vi "WriteValueToQueueDisplay.vi"(8 "error in (no error)":errorcluster, 11 "XuLyStringUART in":refnum<class "XuLyStringUART.lvclass">) -> (0 "error out":errorcluster, 3 "XuLyStringUART out":refnum<class "XuLyStringUART.lvclass">)   [LabVIEW 2017, in "LibraryGcode.lvlib" / "XuLyStringUART.lvclass"]
uses:
  XuLyStringUART.lvclass
  control/UartCmdQueueUpdate.ctl
panel:
  in  "Command":T1
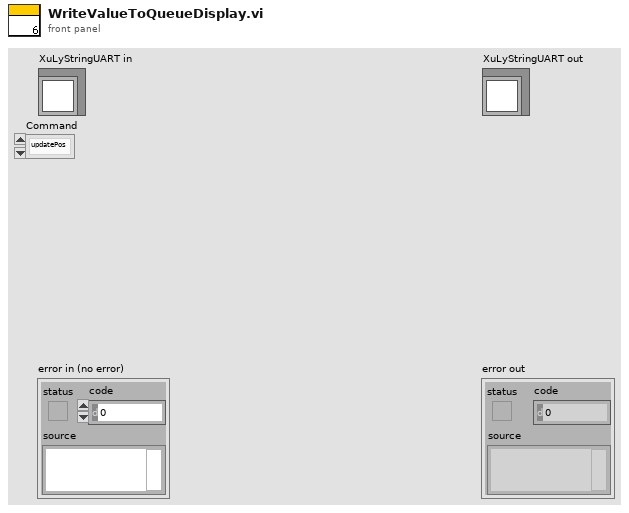
[diagram p1: front panel]
types:
  T1 = typedef "UartCmdQueueUpdate.ctl" = enum16{"updatePos", "UpdateConfigAccel", "UpdateConfigFeed", "UpdateConfigUnit", "UpdateConfigStartAccel"}
  T2 = cluster{"Command":T1, "POS":cluster{"X":dbl, "Y":dbl, "Z":dbl}, "DEGREES":cluster{"X":dbl, "Y":dbl}}
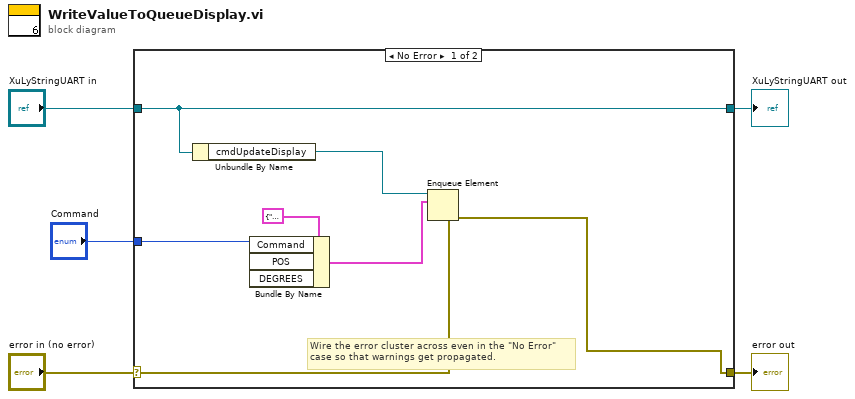
[diagram p0: block diagram]
diagram:
  n1 = case shown="No Error" "error in (no error)" {
    selector: "error in (no error)" -> [w11 w14]
    tunnel: [w10 w14] -> w4
    tunnel: [w12 w13] -> w2
    tunnel: "XuLyStringUART in" -> [w12 w13]
    tunnel: "Command" -> [w6 _]
    frame No Error {
      # "Wire the error cluster across even in the \"No Error\"\ncase so that warnings get propagated."
      n2 = Unbundle By Name(w12) -> ("cmdUpdateDisplay"=w9:refnum<queue>)
      n3 = Bundle By Name(cluster=T2 {"Command"=enum."updatePos", "POS"={"X"=0.0, "Y"=0.0, "Z"=0.0}, "DEGREES"={"X"=0.0, "Y"=0.0}} ("element"), "Command"=w6) -> (w7:T2)  [unwired: 2 in]
      n4 = Enqueue Element(queue=w9, element=w7, error in (no error)=w11) -> (error out=w10:errorcluster)  [unwired: 1 in, 2 out]
    }
    frame Error {
    }
  }
  "error out" <- w4
  "XuLyStringUART out" <- w2
